vi "Initialize Attributes.vi"(8 "error in (no error)":errorcluster, 10 "Attribute Data":variant, 11 "CS++PPG in":refnum<class "CS++PPG.lvclass">) -> (0 "error out":errorcluster, 2 "Found?":bool, 3 "CS++PPG out":refnum<class "CS++PPG.lvclass">)   [LabVIEW 2015, in "CS++PPG.lvlib" / "CS++PPG.lvclass"]
doc: "Initialize object attribute.\n\nUnique resources should be allocated elsewhere!"
uses:
  CS++PPG.lvclass
  PV-Enum.ctl
  CSPP_Core/Classes/CS++ProcessVariables/ProcessVariable/PV.lvclass
  CSPP_Core/Actors/CS++BaseActor/CS++BaseActor.lvclass/CS++BaseActor.ctl
  CSPP_Core/Classes/CS++ProcessVariables/ProcessVariable/PV.lvclass/PV.ctl
  CS++PPG.lvclass/CS++PPG.ctl
  CSPP_Core/Classes/CS++ProcessVariables/ProcessVariable/Write PV URL.vi
  CSPP_Core/Classes/CS++ProcessVariables/ProcessVariable/Write Type Descriptor.vi
  <vilib>/Utility/error.llb/Error Cluster From Error Code.vi
  CSPP_Core/Actors/CS++DeviceActor/CS++DeviceActor.lvclass
  CSPP_Core/Classes/CS++BaseClasses/Factory/CS++Factory.lvclass
  CSPP_Core/Actors/CS++BaseActor/CS++BaseActor.lvclass
  CSPP_Core/Classes/CS++ProcessVariables/CS++ProcessVariables.lvlib
panel:
  in  "PV-Enum":T1
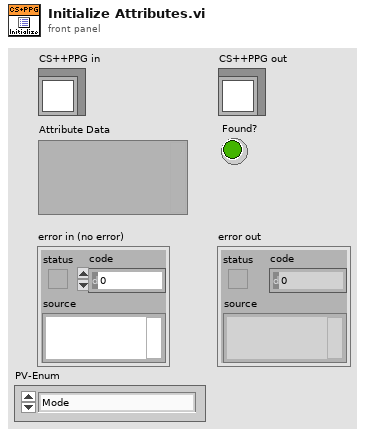
[diagram p1: front panel]
types:
  T1 = typedef "CS++PPG.lvlib/CS++PPG.lvclass/PV-Enum.ctl" = enum16{"Mode"}
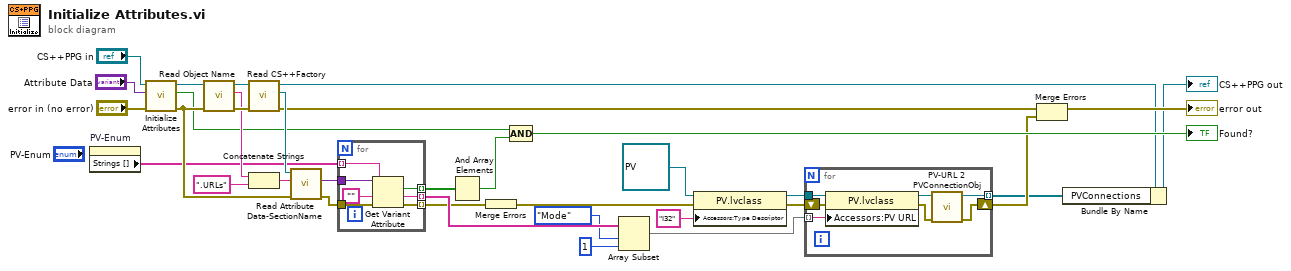
[diagram p0: block diagram]
diagram:
  n1 = property on="PV-Enum" class="Enum (strict)"() -> ("Strings []"=w21:string[])  [unwired: 2 in, 2 out]
  n2 = call-parent "Initialize Attributes.vi"("error in (no error)"="error in (no error)", "Attribute Data"="Attribute Data", "CS++DeviceActor in"="CS++PPG in") -> ("error out"=w22:errorcluster, "Found?"=w19:bool, "CS++DeviceActor out"=w25:refnum<class "CS++PPG.lvclass">)  [unwired: 6 in]
  n3 = call "Read Object Name.vi"("error in (no error)"=w22, "CS++BaseActor in"=w25) -> ("error out"=w30:errorcluster, "Object Name"=w28:string, "CS++BaseActor out"=w31:refnum<class "CS++PPG.lvclass">)  [unwired: 7 in]
  n4 = call "Read CS++Factory.vi"("error in (no error)"=w30, "CS++BaseActor in"=w31) -> ("error out"=w6:errorcluster, "CS++Factory"=w27:refnum<class "CS++Factory.lvclass">, "CS++BaseActor out"=w3:refnum<class "CS++PPG.lvclass">)  [unwired: 7 in]
  n5 = Concatenate Strings(w28, ".URLs" ("string")) -> (w24:string)
  n6 = call-dynamic "Read Attribute Data-SectionName.vi"("error in (no error)"=w22, "Object Name"=w24, "CS++Factory in"=w27) -> ("error out"=w23:errorcluster, "Attribute Data"=w29:variant)  [unwired: 6 in, 1 out]
  n7 = for {
    tunnel: w29 -> [w40]
    tunnel: w23 -> [w39]
    tunnel: w21 -> [w38] mode=indexing
    tunnel: [w37] -> w20 mode=indexing
    tunnel: [w36] -> w10 mode=indexing
    tunnel: [w35] -> w8 mode=indexing
    n8 = Get Variant Attribute(Variant=w40, name=w38, default value (empty Variant)="", error in=w39) -> (found=w37:bool, value=w36:string, error out=w35:errorcluster)  [unwired: 1 out]
  }
  n9 = And Array Elements(Boolean array=w20) -> (logical AND=w17:bool)
  n10 = Merge Errors(w8) -> (w7:errorcluster)
  n11 = Compound Arithmetic op=AND(w19, w17) -> (→"Found?":bool)
  n12 = Array Subset(array=w10, index=PV-Enum."Mode" ("PV-Enum"), length=1) -> (w16:string[])
  n13 = property class="PV.lvclass"(reference=refnum<class "PV.lvclass"> refnum ("CS++ProcessVariables.lvlib:PV.lvclass"), error in=w7, "Accessors:Type Descriptor"="I32" ("Type Descriptor")) -> (reference out=w14:refnum<class "PV.lvclass">, error out=w13:errorcluster)
  n14 = for {
    tunnel: w14 -> [w47]
    tunnel: w16 -> [w46] mode=indexing
    tunnel: [w45] -> w1 mode=indexing
    shift-right: [w44] -> w4
    shift-left: w13 -> [w42]
    n15 = property class="PV.lvclass"(reference=w47, error in=w42, "Accessors:PV URL"=w46) -> (reference out=w48:refnum<class "PV.lvclass">, error out=w43:errorcluster)
    n16 = call "PV-URL 2 PVConnectionObj.vi"("Error In"=w43, "PV"=w48) -> ("Error Out"=w44:errorcluster, "PVConnection"=w45:refnum<class "PVConnection.lvclass">)  [unwired: 7 in, 1 out]
  }
  n17 = Merge Errors(w6, w4) -> (→"error out":errorcluster)
  n18 = Bundle By Name(cluster=w3, "PVConnections"=w1) -> (→"CS++PPG out":refnum<class "CS++PPG.lvclass">)
